vi "Phasor Check Gate Calculation Type v2.vi"(8 "Error In":errorcluster, 10 "Gates Definitions in":T1={"First Gate: t1"=0.0, "Gate Width: W"=0.0, "Gate Step: d"=0.0, "# Gates: G"=0.0, "Use Gate Center"=FALSE, "Frames/Image: F"=0, "Gates/Frame: L"=0, "Bits/Frame: q"=0, "Multiplicity: p"=0, "Gate Type"=enum."Square", "Gate Edge s"=0.0, "Gate Top Slope"=0.0, "Reversed Sawtooth?"=FALSE, "Computation"=FALSE, "User-defined Gate"={"X Array"=[], "Y Array"=[]}, "Tolerance"=0.0, "Integration"=enum."Item 0", "# Steps"=50.0, "Type of User-defined Function"=enum."Gate"}, 11 "Phasor Calculation Type in":T4) -> (0 "Error Out":errorcluster, 2 "Gates Definitions out":T1={"First Gate: t1"=0.0, "Gate Width: W"=0.0, "Gate Step: d"=0.0, "# Gates: G"=0.0, "Use Gate Center"=FALSE, "Frames/Image: F"=0, "Gates/Frame: L"=0, "Bits/Frame: q"=0, "Multiplicity: p"=0, "Gate Type"=enum."Square", "Gate Edge s"=0.0, "Gate Top Slope"=0.0, "Reversed Sawtooth?"=FALSE, "Computation"=FALSE, "User-defined Gate"={"X Array"=[], "Y Array"=[]}, "Tolerance"=0.0, "Integration"=enum."Item 0", "# Steps"=50.0, "Type of User-defined Function"=enum."Gate"}, 3 "Phasor Calculation Type out":T4)   [LabVIEW 2021, in "Phasor.lvlib"]
uses:
  Phasor.lvlib
  Phasor Calculation Type.ctl
  Phasor Gate Definitions.ctl
  Phasor Gate Type.ctl
  Graphs/XY Graph/XY Plot Data.ctl
  Graphs/XY Graph/XY Graph Add-Ons.lvlib
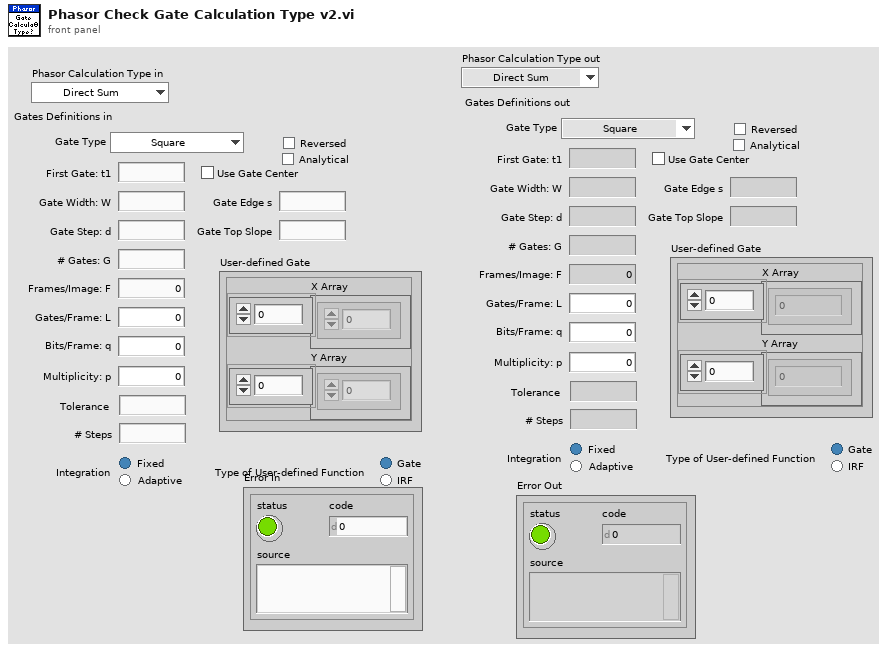
[diagram p1: front panel]
types:
  T1 = typedef "Phasor.lvlib/Phasor Gate Definitions.ctl" = cluster{"First Gate: t1":ext, "Gate Width: W":ext, "Gate Step: d":ext, "# Gates: G":ext, "Use Gate Center":bool, "Frames/Image: F":i32, "Gates/Frame: L":i32, "Bits/Frame: q":i32, "Multiplicity: p":i32, "Gate Type":T2, "Gate Edge s":ext, "Gate Top Slope":ext, "Reversed Sawtooth?":bool, "Computation":bool, "User-defined Gate":T3, "Tolerance":ext, "Integration":enum32{"Item 0", "Item 1"}, "# Steps":ext, "Type of User-defined Function":enum32{"Gate", "IRF"}}
  T2 = typedef "Phasor.lvlib/Phasor Gate Type.ctl" = enum16{"Square", "Finite Edge Square", "Finite Edge, Tilted Top Square", "Triangle", "Sawtooth", "User-defined"}
  T3 = typedef "XY Graph Add-Ons.lvlib/XY Plot Data.ctl" = cluster{"X Array":dbl[], "Y Array":dbl[]}
  T4 = typedef "Phasor.lvlib/Phasor Calculation Type.ctl" = enum16{"Direct Sum", "Analytical Formula"}
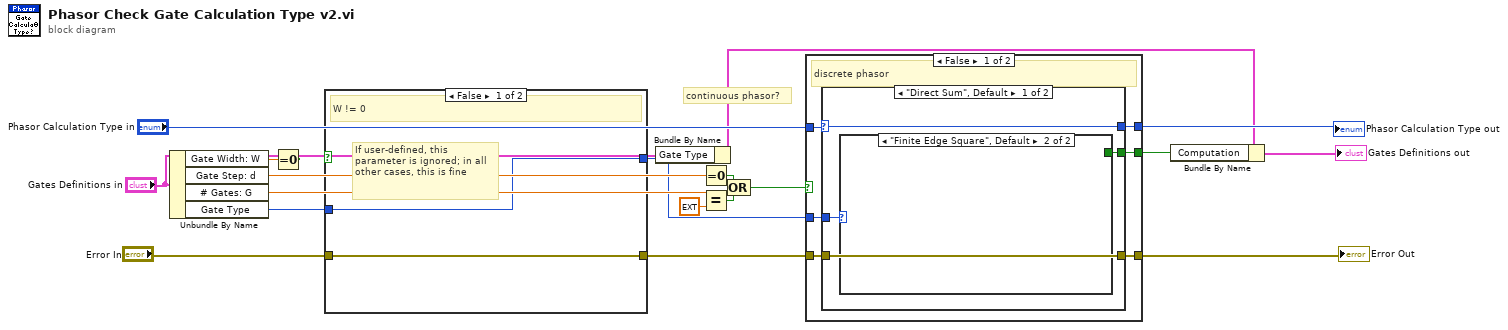
[diagram p0: block diagram]
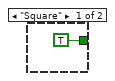
[diagram p2: hidden frame]
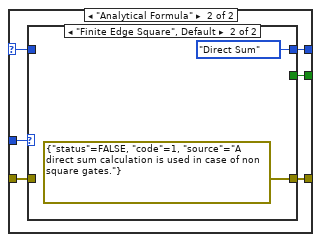
[diagram p3: hidden frame]
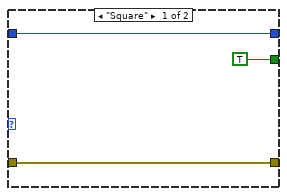
[diagram p4: hidden frame]
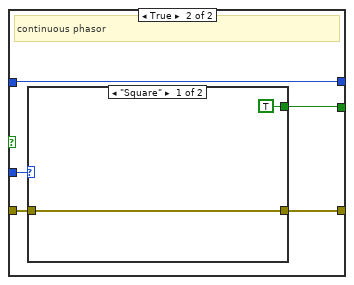
[diagram p5: hidden frame]
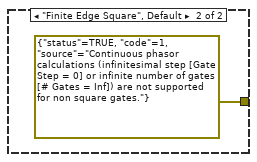
[diagram p6: hidden frame]
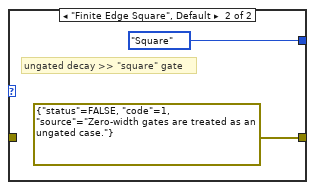
[diagram p8: hidden frame]
diagram:
  # "continuous phasor?"
  n1 = Unbundle By Name("Gates Definitions in") -> ("Gate Width: W"=w14:ext, "Gate Step: d"=w19:ext, "# Gates: G"=w17:ext, "Gate Type"=w11:T2)
  n2 = Equal To 0?(x=w14) -> (x = 0?=w12:bool)
  n3 = case shown="False" w12 {
    tunnel: w11 -> [w21 w25]
    tunnel: [w21 w24] -> w7
    tunnel: [w20 w23] -> w9
    tunnel: "Error In" -> [w20 w22]
    frame False {
      # "If user-defined, this parameter is ignored; in all other cases, this is fine"
      # "W != 0"
    }
    frame True {
      # "W = 0"
      n4 = case shown="\"Square\", \"User-defined\"" w25 {
        selector: w25 -> [w27 _]
        tunnel: [w27 Phasor_Gate_Type."Square" ("Gate Type")] -> w24
        tunnel: [w26 errorcluster {"status"=FALSE, "code"=1, "source"="Zero-width gates are treated as an ungated case."} ("t")] -> w23
        tunnel: w22 -> [w26 _]
        frame "Square", "User-defined" {
          # "These are the only cases where W = 0 is supported"
        }
        frame "Finite Edge Square", Default {
          # "ungated decay >> \"square\" gate"
        }
      }
    }
  }
  n5 = Bundle By Name(cluster="Gates Definitions in", "Gate Type"=w7) -> (w3:T1)
  n6 = Equal To 0?(x=w19) -> (x = 0?=w16:bool)
  n7 = Equal?(x=w17, y=ext inf) -> (x = y?=w15:bool)
  n8 = Compound Arithmetic op=OR(w16, w15) -> (w8:bool)
  n9 = case shown="False" w8 {
    tunnel: w9 -> [w32 w54]
    tunnel: [w31 w56] -> w6
    tunnel: w7 -> [w34 w55]
    tunnel: "Phasor Calculation Type in" -> [w35 w53]
    tunnel: [w33 w53] -> w4
    tunnel: [w30 w52] -> w1
    frame False {
      # "discrete phasor"
      n10 = case shown="\"Direct Sum\", Default" w35 {
        selector: w35 -> [w39 w45]
        tunnel: w34 -> [w37 w46]
        tunnel: [w39 w44] -> w33
        tunnel: w32 -> [w38 w43]
        tunnel: [w38 w42] -> w31
        tunnel: [w36 w41] -> w30
        frame "Direct Sum", Default {
          n11 = case shown="\"Finite Edge Square\", Default" w37 {
            tunnel: [TRUE ("Computation") _] -> w36
            frame "Square" {
            }
            frame "Finite Edge Square", Default {
            }
          }
        }
        frame "Analytical Formula" {
          n12 = case shown="\"Finite Edge Square\", Default" w46 {
            tunnel: w45 -> [w49 _]
            tunnel: [w49 Phasor_Calculation_Type."Direct Sum" ("Phasor Calculation Type in")] -> w44
            tunnel: w43 -> [w48 _]
            tunnel: [w48 errorcluster {"status"=FALSE, "code"=1, "source"="A direct sum calculation is used in case of non square gates."} ("t")] -> w42
            tunnel: [TRUE ("Computation") _] -> w41
            frame "Square" {
            }
            frame "Finite Edge Square", Default {
            }
          }
        }
      }
    }
    frame True {
      # "continuous phasor"
      n13 = case shown="\"Square\"" w55 {
        tunnel: [w58 errorcluster {"status"=TRUE, "code"=1, "source"="Continuous phasor calculations (infinitesimal step [Gate Step = 0] or infinite number of gates [# Gates = Inf]) are not supported for non square gates."} ("t")] -> w56
        tunnel: w54 -> [w58 _]
        tunnel: [TRUE ("Computation") _] -> w52
        frame "Square" {
        }
        frame "Finite Edge Square", Default {
        }
      }
    }
  }
  "Phasor Calculation Type out" <- w4
  "Error Out" <- w6
  n14 = Bundle By Name(cluster=w3, "Computation"=w1) -> (→"Gates Definitions out":T1)
